vi "GT Pvt Percent Calculate.vi"(0 "cardNum":i16, 1 "pPercent":dbl, 2 "pVel":dbl, 5 "n":i32, 7 "pTime":dbl, 9 "pPos":dbl, 11 "error in (no error)":errorcluster caption="错误输入（无错误）", 12 "velBegin":dbl) -> (3 "pPercent out":dbl, 4 "pVel out":dbl, 6 "function return":i16, 8 "pTime out":dbl, 10 "pPos out":dbl, 15 "error out":errorcluster caption="错误输出")   [LabVIEW 2020, in "gts.lvlib"]
doc: "GT_API GT_PvtPercentCalculate(short cardNum,long n,double *pTime,double *pPos,double *pPercent,double velBegin,double *pVel);"
uses:
  gts.lvlib
  dll/32bit/multi_card/gts.dll
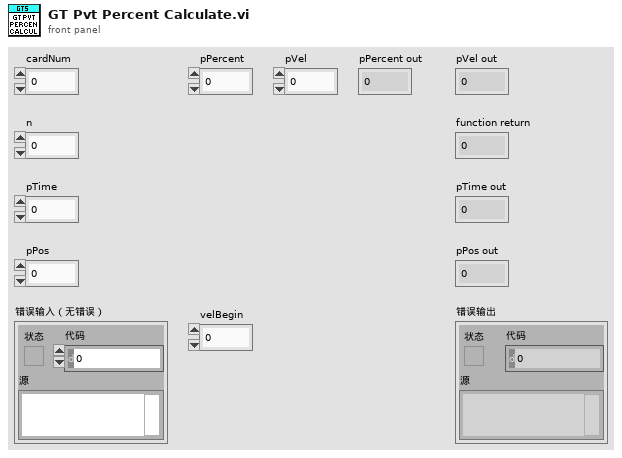
[diagram p1: front panel]
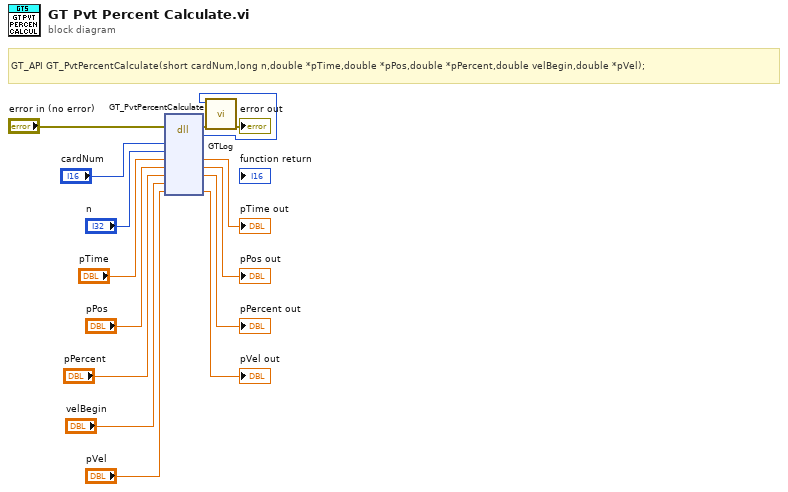
[diagram p0: block diagram]
diagram:
  # "GT_API GT_PvtPercentCalculate(short cardNum,long n,double *pTime,double *pPos,double *pPercent,double velBegin,double *pVel);"
  n1 = dll-call lib="C:/1228/dll/32bit/multi_card/gts.dll" fn="GT_PvtPercentCalculate"(error in="error in (no error)", "cardNum"="cardNum", "n"="n", "pTime"="pTime", "pPos"="pPos", "pPercent"="pPercent", "velBegin"="velBegin", "pVel"="pVel") -> (error out=w3:errorcluster, w1:i16, "pTime"=→"pTime out":dbl, "pPos"=→"pPos out":dbl, "pPercent"=→"pPercent out":dbl, "pVel"=→"pVel out":dbl)  [unwired: 5 in, 1 out]
  n2 = call "GTLog.vi"("error in (no error)"=w3, "Numeric"=w1) -> ("error out"=→"error out":errorcluster)  [unwired: 9 in]
